vi "costo + product.vi"(4 "Inventario":dbl, 5 "Credito":dbl, 6 "Boolean":bool, 7 "Soda?":bool, 8 "Indice":i32, 9 "Costo":dbl, 10 "Producto":string, 11 "Message Enqueuer in":refnum<class "Message Enqueuer.lvclass">) -> (1 "Numeric 2":dbl, 2 "Numeric":dbl, 3 "String":string)   [LabVIEW 2020, in "UI Actor.lvlib" / "UI Actor.lvclass"]
uses:
  UI Actor.lvclass
  <vilib>/ActorFramework/Message Enqueuer/Message Enqueuer.lvclass
  Nestle Actor Messages/Update inventary Msg/Update inventary Msg.lvclass/Update inventary Msg.ctl
  <vilib>/ActorFramework/Message Enqueuer/Message Enqueuer.lvclass/Message Enqueuer.ctl
  Soda Actor Messages/Update Inventary Msg/Update Inventary Msg.lvclass/Update Inventary Msg.ctl
  <vilib>/ActorFramework/Message Enqueuer/Enqueue.vi
  Nestle Actor Messages/Update inventary Msg/Update inventary Msg.lvclass
  C:/Program Files (x86)/National Instruments/LabVIEW 2020/vi.lib/ActorFramework/Message/Message.lvclass
  Soda Actor Messages/Update Inventary Msg/Update Inventary Msg.lvclass
  <vilib>/ActorFramework/Message Priority Queue/Priority Enqueue.vi
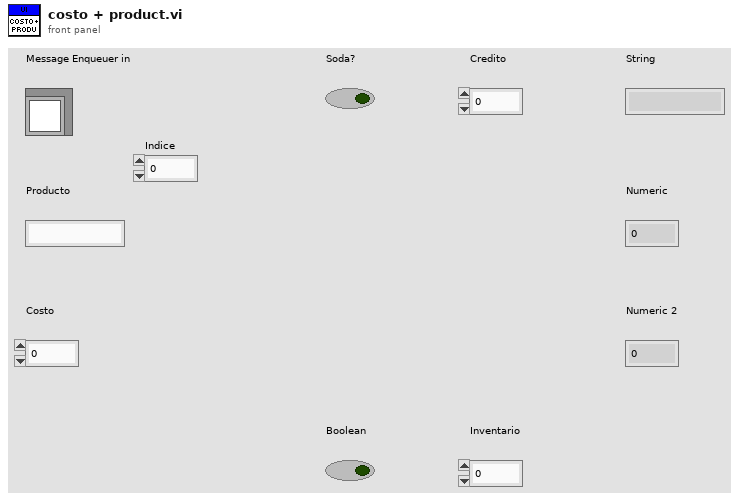
[diagram p1: front panel]
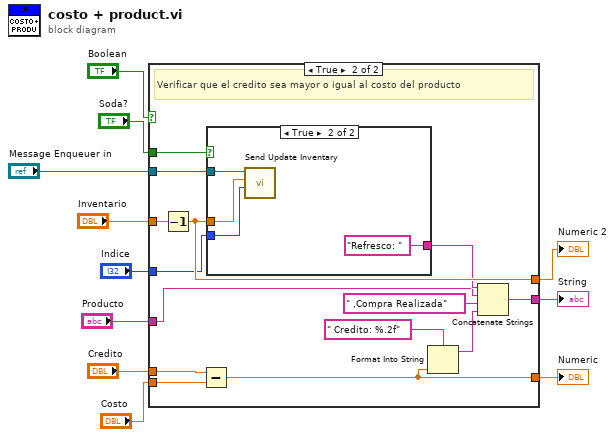
[diagram p0: block diagram]
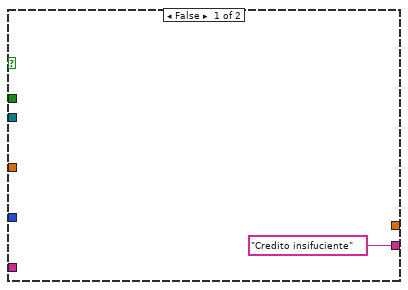
[diagram p2: hidden frame]
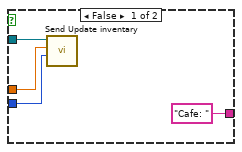
[diagram p3: hidden frame]
diagram:
  n1 = case shown="True" "Boolean" {
    tunnel: "Producto" -> [_ w14]
    tunnel: "Soda?" -> [_ w26]
    tunnel: "Credito" -> [_ w22]
    tunnel: "Costo" -> [_ w21]
    tunnel: ["Credito insifuciente" w20] -> w7
    tunnel: "Inventario" -> [_ w19]
    tunnel: "Message Enqueuer in" -> [_ w18]
    tunnel: [_ w17] -> w10
    tunnel: [_ w16] -> w11
    tunnel: "Indice" -> [_ w13]
    frame False {
    }
    frame True {
      # "Verificar que el credito sea mayor o igual al costo del producto"
      n2 = Decrement(x=w19) -> (x-1=w17:dbl)
      n3 = Subtract(x=w22, y=w21) -> (x-y=w16:dbl)
      n4 = case shown="True" w26 {
        tunnel: ["Cafe: " ("string") "Refresco: " ("string")] -> w15
        tunnel: w17 -> [w28 w33]
        tunnel: w18 -> [w29 w32]
        tunnel: w13 -> [w27 w31]
        frame False {
          n5 = call "Send Update inventary.vi"("Indice"=w27, "Inventario"=w28, "Message Enqueuer"=w29) -> ()  [unwired: 7 in, 2 out]
        }
        frame True {
          n6 = call "Send Update Inventary.vi"("Indice"=w31, "Inventario"=w33, "Message Enqueuer"=w32) -> ()  [unwired: 7 in, 2 out]
        }
      }
      n7 = Format Into String(format string=" Credito: %.2f", w16) -> (resulting string=w24:string)  [unwired: 2 in, 1 out]
      n8 = Concatenate Strings(w15, w14, " ,Compra Realizada" ("string"), w24) -> (w20:string)
    }
  }
  "Numeric" <- w11
  "Numeric 2" <- w10
  "String" <- w7
